vi "Actor-Caller.vi"(5 "Initialize-Error Passback":refnum<notifier>, 7 "Enqueuers Passback":refnum<notifier>, 8 "Owner":refnum<vi>, 9 "Actor-Stopped":refnum<user-event>, 10 "Launch":refnum<notifier>, 11 "Actor in":refnum<class "Actor.lvclass">) -> ()   [LabVIEW 2018, in "Scripting.lvlib" / "Actor.lvlib" / "Interface.lvclass"]
uses:
  Interface.lvclass
  Actor.lvclass
  Request-Enqueuers.ctl
  Get State.ctl
  State.ctl
  Stop.ctl
  Actor-Stopped.ctl
  Front-Panel State.ctl
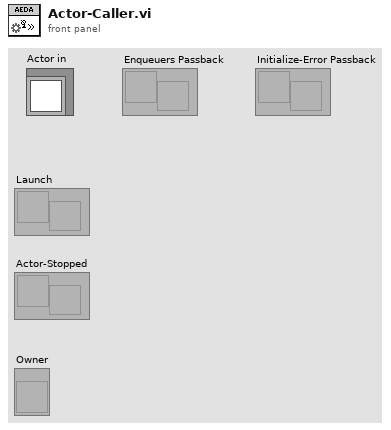
[diagram p1: front panel]
types:
  T1 = typedef "Scripting.lvlib/Actor.lvlib/Interface.lvclass/Actor-Stopped.ctl" = cluster{"Final State":refnum<class "Actor.lvclass">, "Final Error":errorcluster}
  T2 = typedef "Scripting.lvlib/Actor.lvlib/Actor.lvclass/Request-Enqueuers.ctl" = cluster{"Get State":refnum<user-event>, "Stop":refnum<user-event>}
  T3 = typedef "Scripting.lvlib/Actor.lvlib/Actor.lvclass/API-Requests.ctl" = refnum<event-registration>
  T4 = typedef "Scripting.lvlib/Actor.lvlib/Actor.lvclass/Front-Panel State.ctl" = enum16{"Don't Show", "Show"}
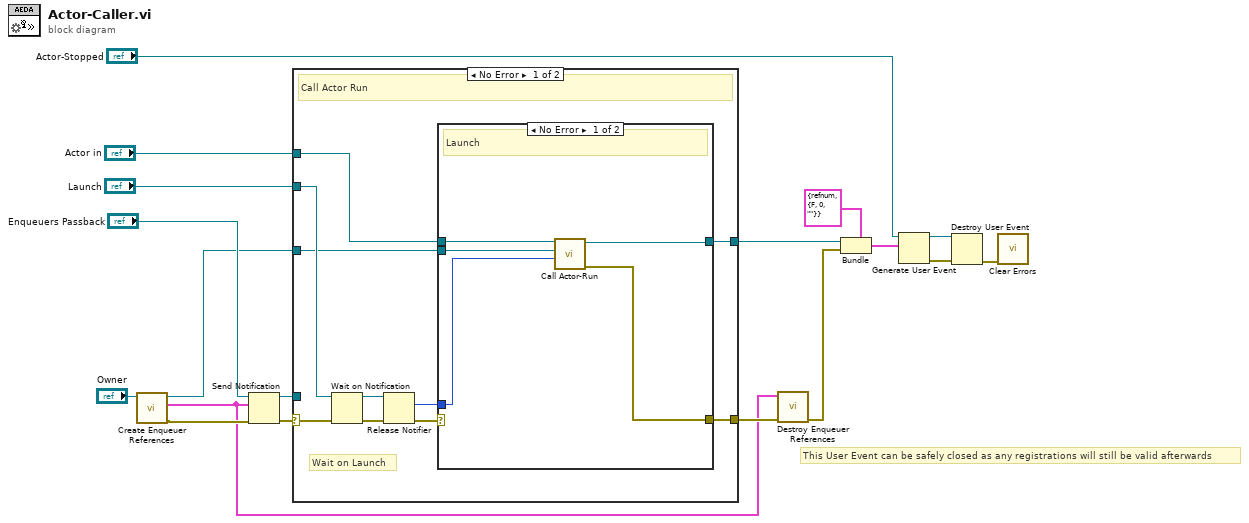
[diagram p0: block diagram]
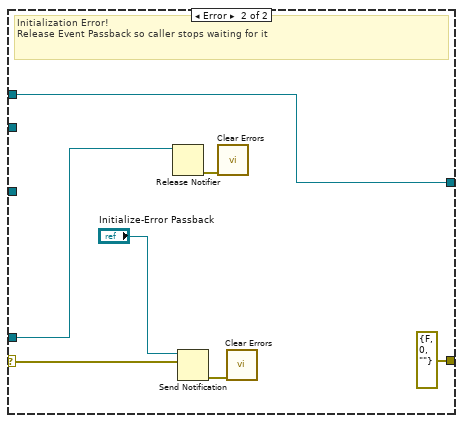
[diagram p3: hidden frame]
diagram:
  # "This User Event can be safely closed as any registrations will still be valid afterwards"
  n1 = call "Create Enqueuer References.vi"("Owner"="Owner") -> ("error out"=w3:errorcluster, "Request-Enqueuers"=w1:T2, "API-Requests"=w4:T3)  [unwired: 8 in]
  n2 = Send Notification(notification=w1, notifier="Enqueuers Passback", error in (no error)=w3) -> (notifier out=w10:refnum<notifier>, error out=w14:errorcluster)
  n3 = case shown="No Error" w14 {
    selector: w14 -> [w26 w37]
    tunnel: "Launch" -> [w28 _]
    tunnel: "Actor in" -> [w27 w41]
    tunnel: [w20 errorcluster {"status"=FALSE, "code"=0, "source"=""} ("error out")] -> w9
    tunnel: [w25 w41] -> w11
    tunnel: w10 -> [_ w40]
    tunnel: w4 -> [w19 _]
    frame No Error {
      # "Wait on Launch"
      # "Call Actor Run"
      n4 = Wait on Notification(notifier=w28, error in (no error)=w26) -> (notifier out=w23:refnum<notifier>, error out=w24:errorcluster)  [unwired: 2 in, 2 out]
      n5 = Release Notifier(notifier=w23, error in (no error)=w24) -> (last notification=w22:T4, error out=w21:errorcluster)  [unwired: 1 in, 1 out]
      n6 = case shown="No Error" w21 {
        tunnel: w27 -> [w33 w34]
        tunnel: [w32 w34] -> w25
        tunnel: [w31 _] -> w20
        tunnel: w22 -> [w30 _]
        tunnel: w19 -> [w29 _]
        frame No Error {
          # "Launch"
          n7 = call "Call Actor-Run.vi"("Front Panel State"=w30, "API-Requests"=w29, "Actor in"=w33) -> ("error out"=w31:errorcluster, "Actor out"=w32:refnum<class "Actor.lvclass">)  [unwired: 7 in]
        }
        frame Error {
          # "Notifier Destroyed Without Launch"
        }
      }
    }
    frame Error {
      # "Initialization Error!\nRelease Event Passback so caller stops waiting for it"
      n8 = Release Notifier(notifier=w40) -> (error out=w39:errorcluster)  [unwired: 2 in, 2 out]
      n9 = Send Notification(notification=w37, notifier="Initialize-Error Passback") -> (error out=w36:errorcluster)  [unwired: 1 in, 1 out]
      n10 = call <vilib>:"Clear Errors.vi"("error in (no error)"=w39) -> ()  [unwired: 5 in, 2 out]
      n11 = call <vilib>:"Clear Errors.vi"("error in (no error)"=w36) -> ()  [unwired: 5 in, 2 out]
    }
  }
  n12 = call "Destroy Enqueuer References.vi"("error in (no error)"=w9, "Requests"=w1) -> ("error out"=w8:errorcluster)  [unwired: 9 in]
  n13 = Bundle(cluster=T1 {"Final State"=refnum, "Final Error"={"status"=FALSE, "code"=0, "source"=""}} ("event data"), "Final State"=w11, "Final Error"=w8) -> (w18:T1)
  n14 = Generate User Event(user event="Actor-Stopped", event data cluster=w18) -> (user event out=w7:refnum<user-event>, error out=w6:errorcluster)  [unwired: 2 in]
  n15 = Destroy User Event(user event=w7, error in=w6) -> (error out=w5:errorcluster)
  n16 = call <vilib>:"Clear Errors.vi"("error in (no error)"=w5) -> ()  [unwired: 5 in, 2 out]
